vi "Read from File.vi"(7 "Channel Direction":string, 8 "error in (no error)":errorcluster, 11 "TXT in":refnum<class "TXT.lvclass">) -> (0 "error out":errorcluster, 2 "Channels":refnum<class "Channel.lvclass">[](array[class]), 3 "TXT out":refnum<class "TXT.lvclass">)   [LabVIEW 2020, in "TXT.lvlib" / "TXT.lvclass"]
uses:
  TXT.lvclass
  built/windows/Channel.lvlibp/Channel.lvclass
  TXT.lvclass/TXT.ctl
  built/windows/ImportExport.lvlibp/ConfigFile/ConfigFile.lvclass
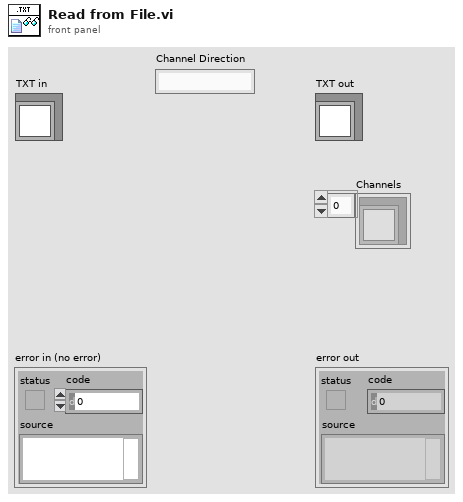
[diagram p1: front panel]
types:
  T1 = typedef "NI_Data Type.lvlib/Data Type.ctl" = enum8{"Invalid Type", "Void", "I8", "I16", "I32", "I64", "U8", "U16", "U32", "U64", "Single Float", "Double Float", "Extended Float", "Single Complex", "Double Complex", "Extended Complex", "Enum U8", "Enum U16", "Enum U32", "Enum U64", "Single Float With Unit", "Double Float With Unit", "Extended Float With Unit", "Single Complex with Unit", "Double Complex with Unit", "Extended Complex with Unit", "Boolean", "String", "Path", "Picture", "Tag", "Array", "Cluster", "Variant", "LV Variant", "Waveform", "Timestamp", "Digital Waveform", "Digital Data", "ExpressData", "Refnum", "External Data", "VI", "Poly VI", "LabVIEW Class Instance", "Fixed Point", "Set Collection", "Map Collection"}
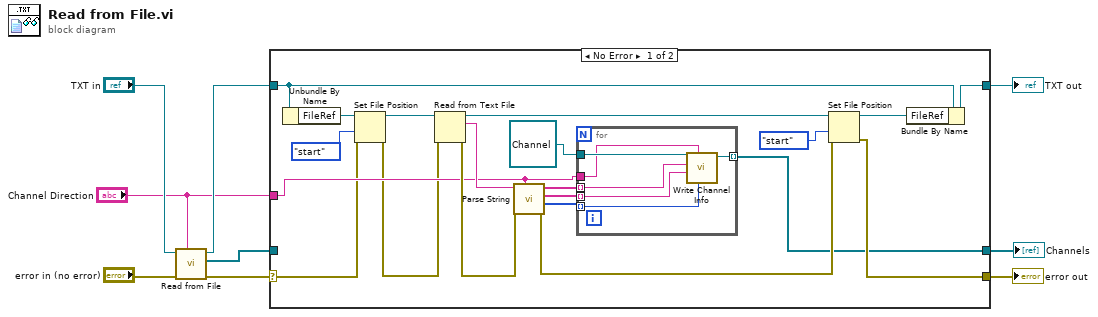
[diagram p0: block diagram]
diagram:
  n1 = call-parent "Read from File.vi"("Channel Direction"="Channel Direction", "error in (no error)"="error in (no error)", "ConfigFile in"="TXT in") -> ("error out"=w6:errorcluster, "Channels"=w3:refnum<class "Channel.lvclass">[], "ConfigFile out"=w4:refnum<class "TXT.lvclass">)  [unwired: 6 in]
  n2 = case shown="No Error" w6 {
    selector: w6 -> [w12 w38]
    tunnel: [w16 w38] -> w9
    tunnel: [w29 w37] -> w8
    tunnel: w4 -> [w26 w37]
    tunnel: [w15 w36] -> w1
    tunnel: w3 -> [_ w36]
    tunnel: "Channel Direction" -> [w17 _]
    frame No Error {
      n3 = Unbundle By Name(w26) -> ("FileRef"=w14:refnum<file>)
      n4 = Set File Position(refnum=w14, from (0:start)=enum16{"start", "end", "current"}."start", error in=w12) -> (refnum out=w13:refnum<file>, error out=w11:errorcluster)  [unwired: 1 in]
      n5 = Read from Text File(file (use dialog)=w13, error in=w11) -> (refnum out=w28:refnum<file>, text=w22:string, error out=w19:errorcluster)  [unwired: 2 in, 1 out]
      n6 = call "Parse String.vi"("Channel Direction"=w17, "error in (no error)"=w19, "Read String"=w22) -> ("error out"=w18:errorcluster, "DataTypes"=w23:T1[], "URLs"=w24:string[], "Name"=w25:string[])  [unwired: 5 in]
      n7 = for {
        tunnel: refnum<class "Channel.lvclass"> refnum ("Channel.lvlibp:Channel.lvclass") -> [w35]
        tunnel: [w34] -> w15 mode=indexing
        tunnel: w25 -> [w32] mode=indexing
        tunnel: w24 -> [w31] mode=indexing
        tunnel: w23 -> [w33] mode=indexing
        tunnel: w17 -> [w30]
        n8 = call "Write Channel Info.vi"("DataType"=w33, "Read or Write"=w30, "URL"=w31, "Name"=w32, "Channel in"=w35) -> ("Channel out"=w34:refnum<class "Channel.lvclass">)  [unwired: 5 in, 1 out]
      }
      n9 = Set File Position(refnum=w28, from (0:start)=enum16{"start", "end", "current"}."start", error in=w18) -> (refnum out=w21:refnum<file>, error out=w16:errorcluster)  [unwired: 1 in]
      n10 = Bundle By Name(cluster=w26, "FileRef"=w21) -> (w29:refnum<class "TXT.lvclass">)
    }
    frame Error {
    }
  }
  "error out" <- w9
  "TXT out" <- w8
  "Channels" <- w1
